vi "Test Get Named Ranges of Sheet.vi"(11 "Test Case In":refnum<class "Test Open Xml.lvclass">) -> (0 "error out":errorcluster, 3 "Test Case Out":refnum<class "Test Open Xml.lvclass">)   [LabVIEW 2021, in "Test Open Xml.lvclass"]
uses:
  Test Open Xml.lvclass
  C:/Program Files/National Instruments/LabVIEW 2025/vi.lib/Astemes/LUnit/Test Case.lvclass
  <vilib>/Astemes/LUnit/Test Case.lvclass/Test Case.ctl
  <vilib>/Astemes/LUnit/Core/LUnit Test Case/Private/Append Fail Result.vi
  <vilib>/Astemes/LUnit/Core/LUnit Test Case/Private/Append Pass Result.vi
  <vilib>/Astemes/LUnit/Core/LUnit Test Case/Private/Run In UI.vi
  <vilib>/Utility/error.llb/Clear Errors.vi
  Source/Open Xml.lvlib
  <vilib>/Astemes/LUnit/Test Case.lvclass
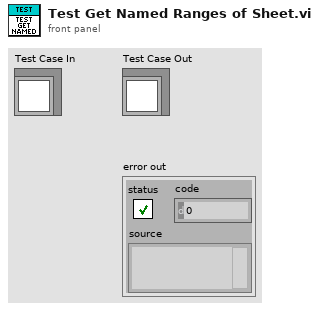
[diagram p1: front panel]
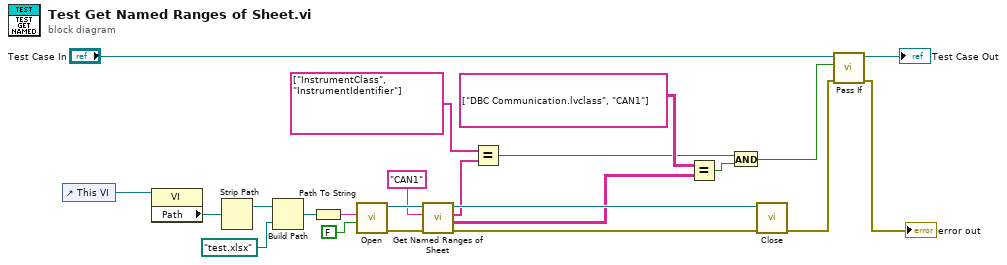
[diagram p0: block diagram]
diagram:
  n1 = control-ref of="This VI"() -> (w20:refnum<vi>)
  n2 = property class="VI"(reference=w20) -> ("Path"=w19:path)  [unwired: 1 in, 2 out]
  n3 = Strip Path(path=w19) -> (stripped path=w18:path)  [unwired: 1 out]
  n4 = Build Path(base path=w18, name or relative path=path "test.xlsx") -> (appended path=w16:path)
  n5 = Path To String(path=w16) -> (string=w15:string)
  n6 = call "Open.vi"("isEditable"=FALSE, "Path"=w15) -> ("error out"=w12:errorcluster, "SpreadsheetDocument"=w13:refnum<k24>)  [unwired: 8 in]
  n7 = call "Get Named Ranges of Sheet.vi"("error in"=w12, "Sheet Name"="CAN1", "SpreadsheetDocument"=w13) -> ("error out"=w10:errorcluster, "Cells"=w4:string[][][], "Range Names"=w7:string[], "SpreadsheetDocument out"=w8:refnum<k24>)  [unwired: 5 in]
  n8 = Equal?(x=string[] ["InstrumentClass", "InstrumentIdentifier"] ("Range Names"), y=w7) -> (x = y?=w2:bool)
  n9 = Equal?(x=string[][][] [[["DBC Communication.lvclass"]], [["CAN1"]]] ("Cells"), y=w4) -> (x = y?=w3:bool)
  n10 = And(x=w2, y=w3) -> (x .and. y?=w1:bool)
  n11 = call "Close.vi"("error in"=w10, "SpreadsheetDocument"=w8) -> ("error out"=w9:errorcluster)  [unwired: 9 in]
  n12 = call <vilib>:"Pass If.vi"("error in (no error)"=w9, "Pass?"=w1, "LUnit Test Case In"="Test Case In") -> ("error out"=→"error out":errorcluster, "LUnit Test Case Out"=→"Test Case Out":refnum<class "Test Open Xml.lvclass">)  [unwired: 7 in]
